vi "Get Local XML Path.vi"(8 "Error In":errorcluster, 11 "Project Path":path) -> (0 "Error Out":errorcluster, 2 "Found ?":bool, 3 "XML Path":path, 5 "Custom Device Name":string, 7 "Common Doc Dir":string)   [LabVIEW 2018, in ".LVLIBP CD XML Updater.lvlib" / "Project XML Editor.lvclass"]
uses:
  Project XML Editor.lvclass
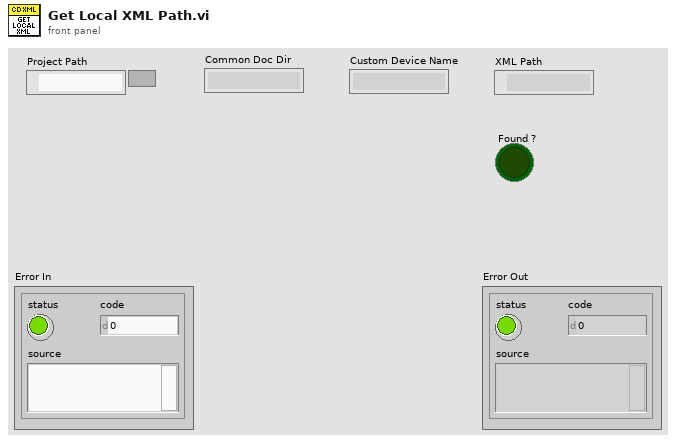
[diagram p1: front panel]
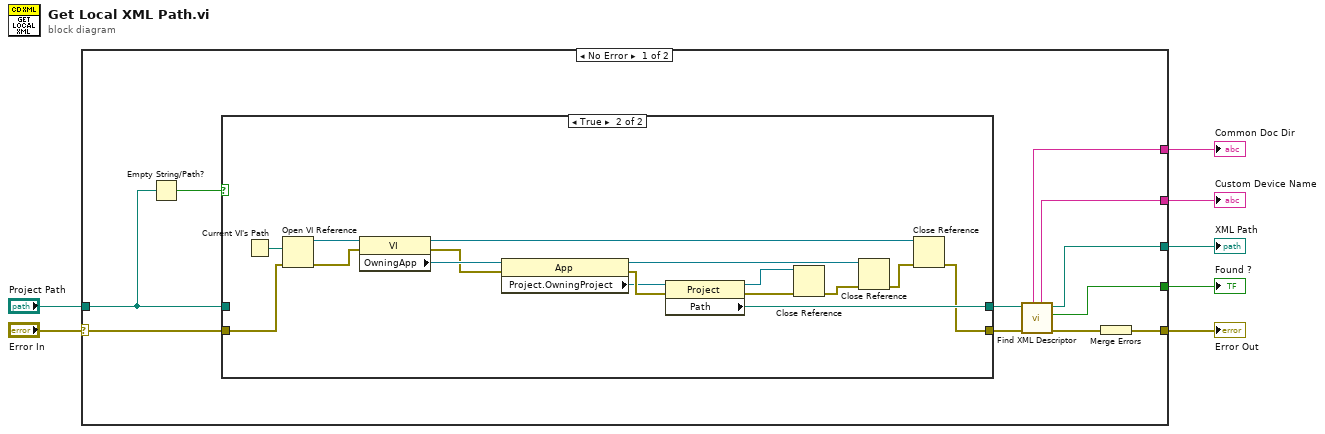
[diagram p0: block diagram]
diagram:
  n1 = case shown="No Error" "Error In" {
    selector: "Error In" -> [w17 w37]
    tunnel: [w15 w37] -> w6
    tunnel: [w14 _] -> w5
    tunnel: [w13 _] -> w4
    tunnel: [w12 _] -> w3
    tunnel: [w11 _] -> w2
    tunnel: "Project Path" -> [w8 _]
    frame No Error {
      n2 = Empty String/Path?(string/path=w8) -> (empty?=w9:bool)
      n3 = case shown="True" w9 {
        tunnel: [w20 w23] -> w18
        tunnel: w17 -> [w19 w22]
        tunnel: [w19 w21] -> w10
        tunnel: w8 -> [w20 _]
        frame False {
        }
        frame True {
          n4 = Current VI's Path() -> (path=w34:path)
          n5 = Open VI Reference(vi path=w34, error in (no error)=w22) -> (vi reference=w33:refnum<vi>, error out=w32:errorcluster)  [unwired: 4 in]
          n6 = property class="VI"(reference=w33, error in=w32) -> (reference out=w29:refnum<vi>, error out=w30:errorcluster, "OwningApp"=w31:refnum<vi>)
          n7 = property class="App"(reference=w31, error in=w30) -> (reference out=w28:refnum<vi>, error out=w36:errorcluster, "Project.OwningProject"=w35:refnum<vi>)
          n8 = property class="Project"(reference=w35, error in=w36) -> (reference out=w27:refnum<vi>, error out=w26:errorcluster, "Path"=w23:path)
          n9 = Close Reference(reference=w27, error in (no error)=w26) -> (error out=w25:errorcluster)
          n10 = Close Reference(reference=w28, error in (no error)=w25) -> (error out=w24:errorcluster)
          n11 = Close Reference(reference=w29, error in (no error)=w24) -> (error out=w21:errorcluster)
        }
      }
      n12 = call "Find XML Descriptor.vi"("error in"=w10, "Project Path"=w18) -> ("error out"=w16:errorcluster, "Found ?"=w13:bool, "XML Path"=w14:path, "Custom Device Name"=w12:string, "Common Doc Dir"=w11:string)  [unwired: 5 in]
      n13 = Merge Errors(w16) -> (w15:errorcluster)
    }
    frame Error {
    }
  }
  "Error Out" <- w6
  "XML Path" <- w5
  "Found ?" <- w4
  "Custom Device Name" <- w3
  "Common Doc Dir" <- w2
